vi "Get BLISS_Select-Make folder.vi"(8 "error in (no error)":errorcluster, 9 "View":string, 10 "BLISS Type":enum16{"Reject Images", "PBQA Images"}(ring), 11 "Data Parameters in in":T1) -> (0 "error out":errorcluster, 1 "File List":string[](array[string]), 2 "Server Name":string, 3 "dup path":path, 4 "Data Parameters out":T1)   [LabVIEW 2020]
uses:
  MC5e Squad_Info.ctl
  MC5e Unit_Status_List.ctl
  MC5e Data_Parameters.ctl
  MC5e Terrain types.ctl
  Location.ctl
  MC5e Unit.ctl
  MC5e Force.ctl
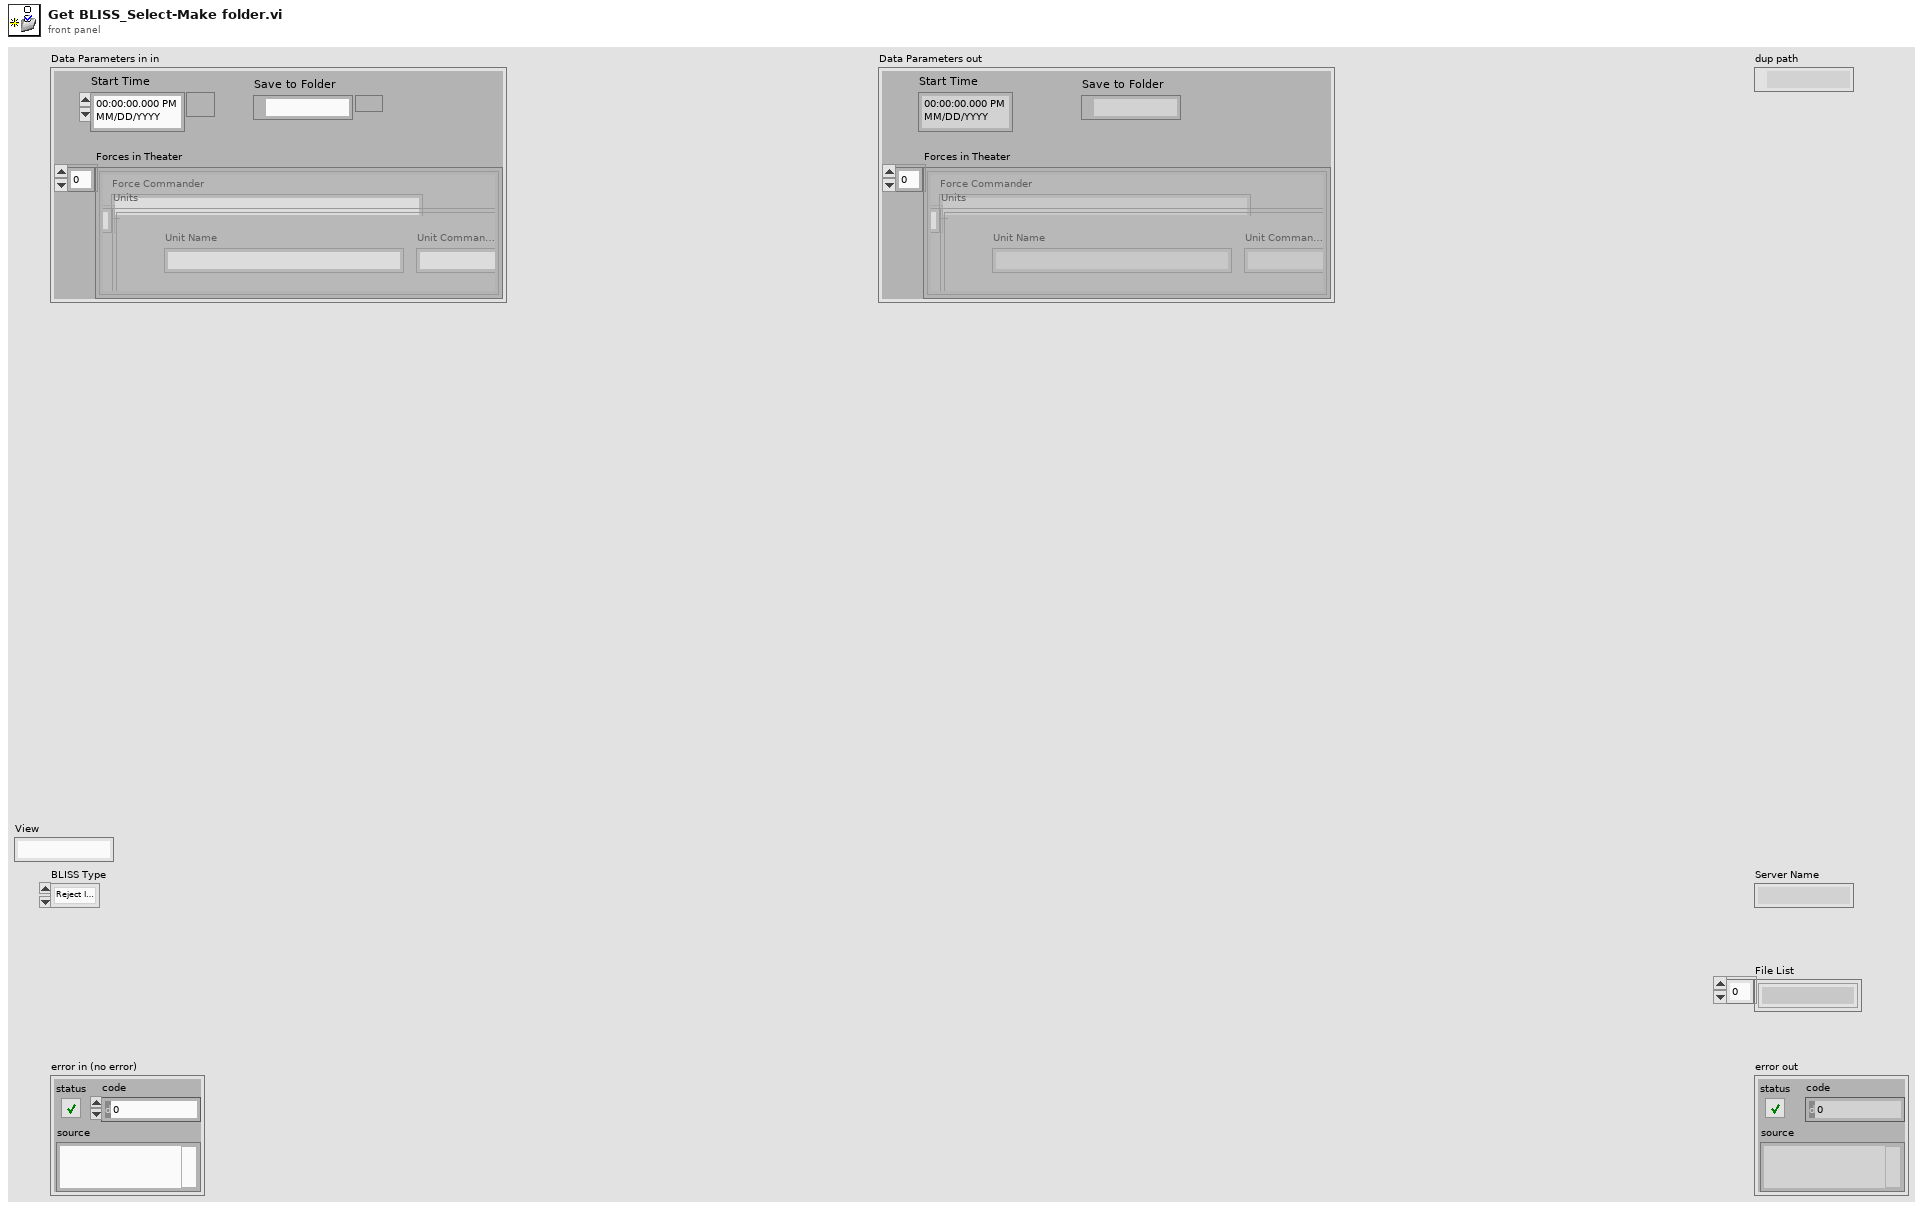
[diagram p1: front panel]
types:
  T1 = typedef "MC5e Data_Parameters.ctl" = cluster{"Start Time":timestamp, "Save to Folder":path, "Forces in Theater":T2[]}
  T2 = typedef "MC5e Force.ctl" = cluster{"Force Commander":string, "Units":T3[]}
  T3 = typedef "MC5e Unit.ctl" = cluster{"Squad List":T4, "Unit Fatigue Level":enum16{"Not Fatigued", "Fatigued", "Seriously Fatigued"}, "Flying Unit":bool, "Mounted Unit":bool, "Difficult Terrain Types":T6, "Full BR":dbl, "Defending from Stronghold":bool, "Speed":dbl, "Capacity %":dbl, "Morale":dbl, "Current BR":dbl, "Location":T7, "Unit Name":string, "Unit Commander":string, "Unit Notes":string}
  T4 = typedef "MC5e Unit_Status_List.ctl" = T5[]
  T5 = typedef "MC5e Squad_Info.ctl" = cluster{"Squad Name":string, "# Soldiers":dbl, "Battle Rating":dbl, "Flying":bool, "Mounted":bool, "Speed":dbl, "Range":dbl, "Morale":dbl, "Token Image":variant, "Max Endurance":dbl, "Current Endurance":dbl, "Difficult Terrain":T6}
  T6 = typedef "MC5e Terrain types.ctl" = cluster{"Artic / snow / ice)":bool, "Coast":bool, "Desert / sand":bool, "Forest / woodland":bool, "Grassland / plains":bool, "Mountain / canyons":bool, "Underdark / caverns":bool, "Acquatic / rivers, lakes, ocean":bool}
  T7 = typedef "Location.ctl" = cluster{"X coordinate":dbl, "Y coordinate":dbl}
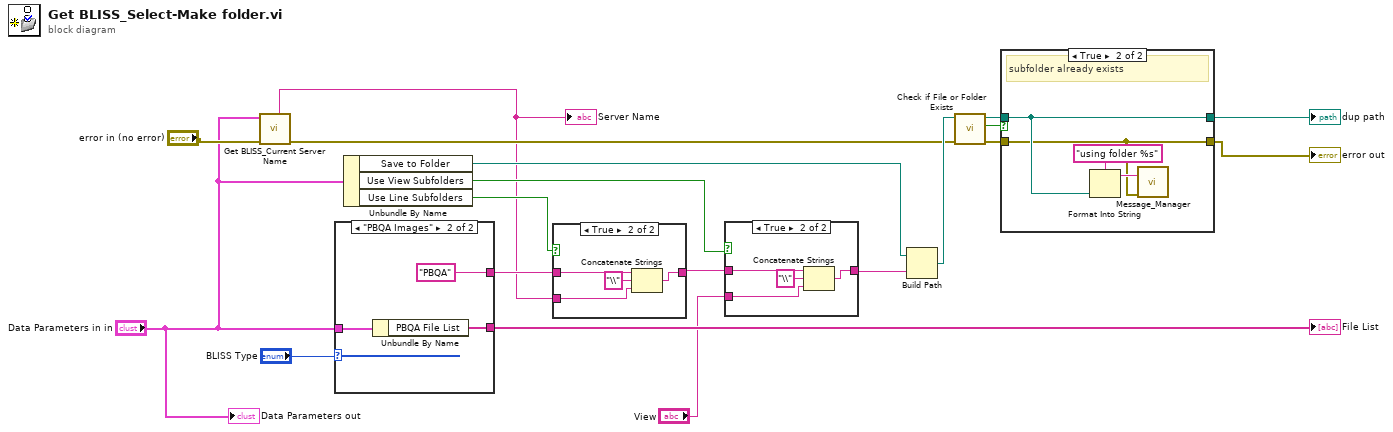
[diagram p0: block diagram]
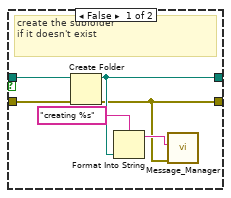
[diagram p4: hidden frame]
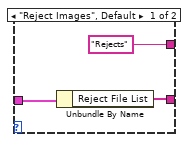
[diagram p5: hidden frame]
diagram:
  n1 = call "Get BLISS_Current Server Name.vi"("error in"="error in (no error)", "Data Parameters in"="Data Parameters in in") -> ("error out"=w11:errorcluster, "Server Name"=w2:string)  [unwired: 6 in, 2 out]
  "Server Name" <- w2
  n2 = case shown="\"PBQA Images\"" "BLISS Type" {
    tunnel: "Data Parameters in in" -> [w20 w23]
    tunnel: [w22 w25] -> w13
    tunnel: ["Rejects" "PBQA"] -> w8
    frame "Reject Images", Default {
      n3 = Unbundle By Name(w20) -> ("Reject File List"=w22:string[])
    }
    frame "PBQA Images" {
      n4 = Unbundle By Name(w23) -> ("PBQA File List"=w25:string[])
    }
  }
  "File List" <- w13
  n5 = Unbundle By Name("Data Parameters in in") -> ("Save to Folder"=w9:path, "Use View Subfolders"=w5:bool, "Use Line Subfolders"=w6:bool)
  n6 = case shown="True" w6 {
    tunnel: w8 -> [w26 w30]
    tunnel: w2 -> [_ w28]
    tunnel: [w26 w27] -> w7
    frame False {
    }
    frame True {
      n7 = Concatenate Strings(w30, "\\" ("string"), w28) -> (w27:string)
    }
  }
  n8 = case shown="True" w5 {
    tunnel: w7 -> [w31 w35]
    tunnel: "View" -> [_ w33]
    tunnel: [w31 w32] -> w3
    frame False {
    }
    frame True {
      n9 = Concatenate Strings(w35, "\\" ("string"), w33) -> (w32:string)
    }
  }
  n10 = Build Path(base path=w9, name or relative path=w3) -> (appended path=w15:path)
  n11 = call <vilib>:"Check if File or Folder Exists.vi"("error in (no error)"=w11, "path"=w15) -> ("error out"=w18:errorcluster, "file or folder exists?"=w16:bool, "dup path"=w17:path)  [unwired: 7 in]
  n12 = case shown="True" w16 {
    tunnel: w17 -> [w41 w44]
    tunnel: w18 -> [w40 w42]
    tunnel: [w36 w42] -> w10
    tunnel: [w37 w44] -> w19
    frame False {
      # "create the subfolder\nif it doesn't exist"
      n13 = Create Folder(path (use dialog)=w41, error in=w40) -> (created path=w37:path, error out=w36:errorcluster)  [unwired: 1 in, 1 out]
      n14 = Format Into String(format string="creating %s", w37) -> (resulting string=w39:string)  [unwired: 2 in, 1 out]
      n15 = call "Message_Manager.vi"("error in"=w36, "New Entry"=w39) -> ()  [unwired: 4 in, 6 out]
    }
    frame True {
      # "subfolder already exists"
      n16 = Format Into String(format string="using folder %s", w44) -> (resulting string=w43:string)  [unwired: 2 in, 1 out]
      n17 = call "Message_Manager.vi"("error in"=w42, "New Entry"=w43) -> ()  [unwired: 4 in, 6 out]
    }
  }
  "error out" <- w10
  "dup path" <- w19
  "Data Parameters out" <- "Data Parameters in in"
